vi "Check-Temperature-values-storage.vi"(7 "Save?":bool, 8 "error in":errorcluster, 9 "Correct. params. ref.":refnum<data-value>, 10 "Temp. params. ref.":refnum<data-value>, 11 "Config. params. ref.":refnum<data-value>) -> (0 "error IO":errorcluster, 3 "Passed?":bool)   [LabVIEW 2013, in "CameraVision.lvlib" / "CV-Storage.lvclass"]
uses:
  CV-Storage.lvclass
  Configuration/CV-Configuration.lvclass
  Temperature/CV-Temperature.lvclass
  Correction/CV-Correction.lvclass
  Correction/CV-Correction.lvclass/CV-Correction.ctl
  Temperature/CV-Temperature.lvclass/CV-Temperature.ctl
  Configuration/CV-Configuration.lvclass/CV-Configuration.ctl
  Configuration/Read Number of cameras.vi
  Temperature/Read Temperature field.vi
  Temperature/Read Temperature value.vi
  Correction/Read 2nd image correlation.vi
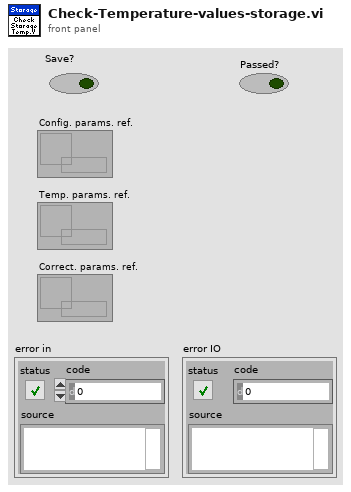
[diagram p1: front panel]
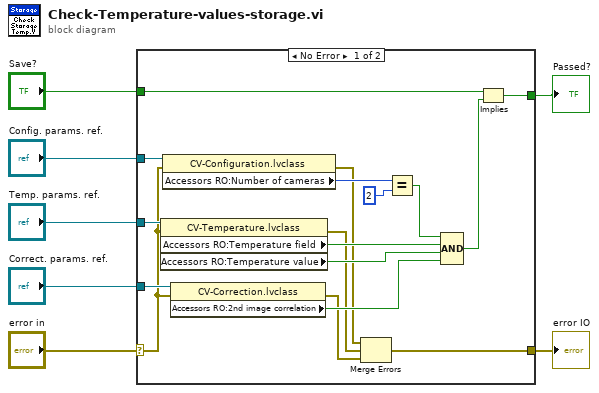
[diagram p0: block diagram]
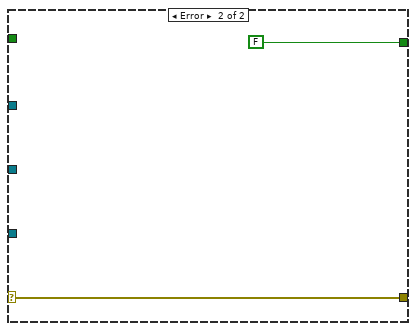
[diagram p2: hidden frame]
diagram:
  n1 = case shown="No Error" "error in" {
    selector: "error in" -> [w12 w25]
    tunnel: "Correct. params. ref." -> [w14 _]
    tunnel: [w8 w25] -> w6
    tunnel: [w23 FALSE] -> w7
    tunnel: "Save?" -> [w22 _]
    tunnel: "Temp. params. ref." -> [w17 _]
    tunnel: "Config. params. ref." -> [w19 _]
    frame No Error {
      n2 = property class="CV-Temperature.lvclass"(reference=w17, error in=w12) -> (error out=w10:errorcluster, "Accessors RO:Temperature field"=w16:bool, "Accessors RO:Temperature value"=w15:bool)  [unwired: 1 out]
      n3 = property class="CV-Configuration.lvclass"(reference=w19, error in=w12) -> (error out=w11:errorcluster, "Accessors RO:Number of cameras"=w18:i32)  [unwired: 1 out]
      n4 = property class="CV-Correction.lvclass"(reference=w14, error in=w12) -> (error out=w9:errorcluster, "Accessors RO:2nd image correlation"=w13:bool)  [unwired: 1 out]
      n5 = Merge Errors(w11, w10, w9) -> (w8:errorcluster)
      n6 = Equal?(x=w18, y=2) -> (x = y?=w20:bool)
      n7 = Compound Arithmetic op=AND(w20, w16, w15, w13) -> (w24:bool)
      n8 = Implies(1:w24, 2:w22) -> (0:w23:bool)
    }
    frame Error {
    }
  }
  "Passed?" <- w7
  "error IO" <- w6
